vi "Init DMA.vi"(8 "error in":errorcluster, 11 "FPGA VI Reference In":refnum<k20>) -> (0 "error out":errorcluster, 3 "FPGA VI Reference Out":refnum<k20>)   [LabVIEW 2014]
doc: "This subVI initializes the FPGA VI. In particular, DMAs are initialized."
uses:
  <vilib>/rvi/interface/common/niFpgaWaitOnOcc.vi
  <vilib>/Utility/error.llb/Error Cluster From Error Code.vi
  <vilib>/rvi/interface/nirviMethod/nirviMethod.xnode
  <vilib>/FPGAPlugInAG/Dynamic/niLvFpga_ConfigureFifo_Dynamic.vi
  <vilib>/rvi/errors/niLvFpgaMergeErrorWithErrorCode.vi
  <vilib>/FPGAPlugInAG/Dynamic/niLvFpga_StartFifo_Dynamic.vi
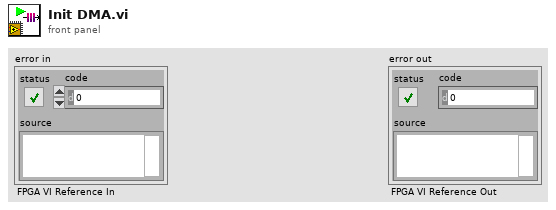
[diagram p1: front panel]
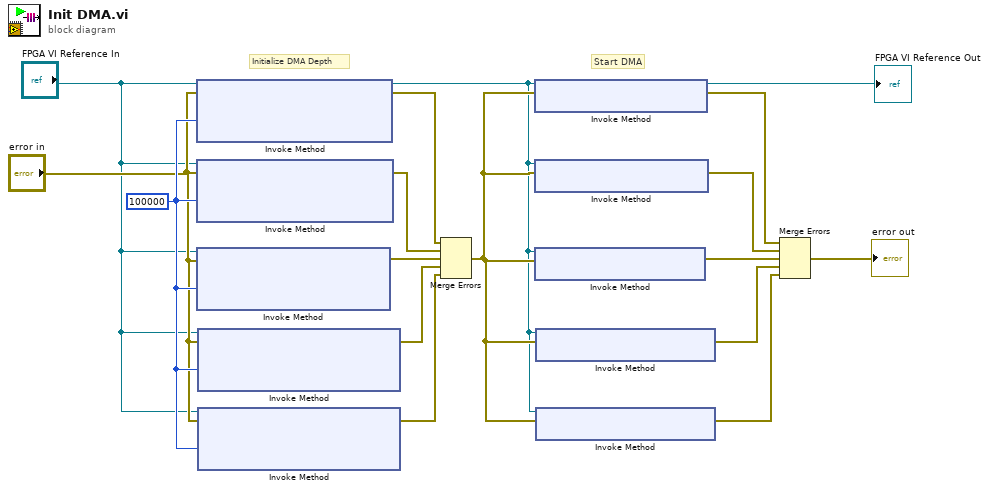
[diagram p0: block diagram]
diagram:
  w17 = u32 100000 ("Requested Depth")
  # "Start DMA"
  # "Initialize DMA Depth"
  n1 = xnode "Invoke Method"("FPGA VI Reference In"="FPGA VI Reference In", "error in"="error in", "Requested Depth"=w17) -> ("FPGA VI Reference Out"=w10:refnum<k20>, "error out"=w16:errorcluster)  [unwired: 1 out]
  n2 = xnode "Invoke Method"("FPGA VI Reference In"="FPGA VI Reference In", "error in"="error in", "Requested Depth"=w17) -> ("error out"=w15:errorcluster)  [unwired: 2 out]
  n3 = xnode "Invoke Method"("FPGA VI Reference In"="FPGA VI Reference In", "error in"="error in", "Requested Depth"=w17) -> ("error out"=w14:errorcluster)  [unwired: 2 out]
  n4 = xnode "Invoke Method"("FPGA VI Reference In"="FPGA VI Reference In", "error in"="error in", "Requested Depth"=w17) -> ("error out"=w13:errorcluster)  [unwired: 2 out]
  n5 = xnode "Invoke Method"("FPGA VI Reference In"="FPGA VI Reference In", "error in"="error in", "Requested Depth"=w17) -> ("error out"=w12:errorcluster)  [unwired: 2 out]
  n6 = Merge Errors(w16, w15, w14, w13, w12) -> (w11:errorcluster)
  n7 = xnode "Invoke Method"("FPGA VI Reference In"=w10, "error in"=w11) -> ("FPGA VI Reference Out"=→"FPGA VI Reference Out":refnum<k20>, "error out"=w9:errorcluster)
  n8 = xnode "Invoke Method"("FPGA VI Reference In"=w10, "error in"=w11) -> ("error out"=w8:errorcluster)  [unwired: 1 out]
  n9 = xnode "Invoke Method"("FPGA VI Reference In"=w10, "error in"=w11) -> ("error out"=w7:errorcluster)  [unwired: 1 out]
  n10 = xnode "Invoke Method"("FPGA VI Reference In"=w10, "error in"=w11) -> ("error out"=w6:errorcluster)  [unwired: 1 out]
  n11 = xnode "Invoke Method"("FPGA VI Reference In"=w10, "error in"=w11) -> ("error out"=w5:errorcluster)  [unwired: 1 out]
  n12 = Merge Errors(w9, w8, w7, w6, w5) -> (→"error out":errorcluster)
